vi "Transmit.vi"(8 "error in (no error)":errorcluster, 10 "Transfer Group in":refnum<class "Transfer Group.lvclass">, 11 "UDP Transceiver in":refnum<class "UDP Transceiver.lvclass">) -> (0 "error out":errorcluster, 2 "Transfer Group out":refnum<class "Transfer Group.lvclass">, 3 "UDP Transceiver out":refnum<class "UDP Transceiver.lvclass">)   [LabVIEW 2023, in "UDP.lvlib" / "UDP Transceiver.lvclass"]
uses:
  UDP Transceiver.lvclass
  Users/Public/Documents/National Instruments/NI VeriStand 2023/Custom Devices/Data Sharing Framework/Linux_x64/DSF Core.lvlibp/Classes/Transfer Group/Transfer Group.lvclass
  UDP Transceiver.lvclass/UDP Transceiver.ctl
  Write Datagram to Port.vi
  <vilib>/Utility/error.llb/Clear Errors.vi
  Users/Public/Documents/National Instruments/NI VeriStand 2023/Custom Devices/Data Sharing Framework/Linux_x64/DSF Core.lvlibp/Classes/Transfer/Get Active Buffer.vi
  Users/Public/Documents/National Instruments/NI VeriStand 2023/Custom Devices/Data Sharing Framework/Linux_x64/DSF Core.lvlibp/Classes/Buffer/Get Buffer Size.vi
  Users/Public/Documents/National Instruments/NI VeriStand 2023/Custom Devices/Data Sharing Framework/Linux_x64/DSF Core.lvlibp/Classes/Buffer/Read Buffer.vi
  Users/Public/Documents/National Instruments/NI VeriStand 2023/Custom Devices/Data Sharing Framework/Linux_x64/DSF Core.lvlibp/Classes/Buffer/Read Buffer 1D U8.vi
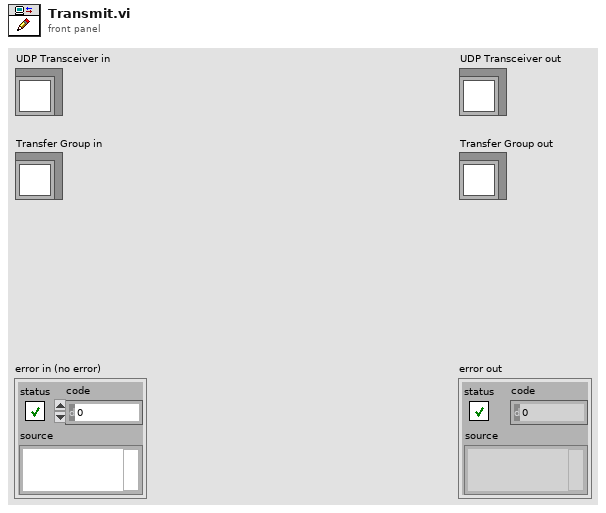
[diagram p1: front panel]
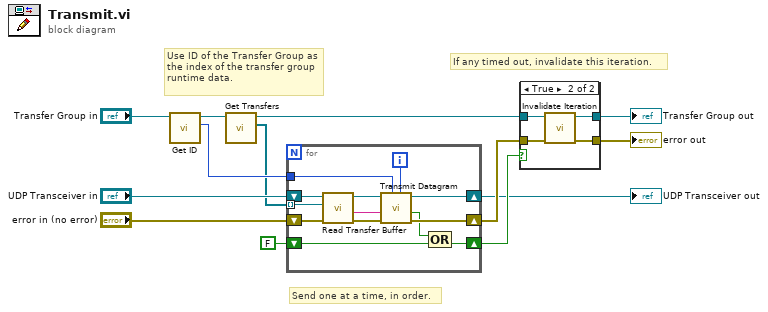
[diagram p0: block diagram]
diagram:
  # "If any timed out, invalidate this iteration."
  # "Send one at a time, in order."
  # "Use ID of the Transfer Group as the index of the transfer group runtime data."
  n1 = call "Get ID.vi"("Transfer Group in"="Transfer Group in") -> ("id"=w13:i32, "Transfer Group out"=w9:refnum<class "Transfer Group.lvclass">)  [unwired: 9 in]
  n2 = call "Get Transfers.vi"("Transfer Group in"=w9) -> ("Transfers"=w1:refnum<class "Transfer.lvclass">[], "Transfer Group out"=w7:refnum<class "Transfer Group.lvclass">)  [unwired: 9 in]
  n3 = for {
    shift-right: [w26] -> w5
    shift-left: "error in (no error)" -> [w18]
    shift-right: [w20] -> w2
    shift-left: "UDP Transceiver in" -> [w19]
    tunnel: w13 -> [w25]
    shift-right: [w21] -> w3
    shift-left: FALSE -> [w23]
    tunnel: w1 -> [w14] mode=indexing
    i -> [w24]
    n4 = call "Read Transfer Buffer.vi"("error in (no error)"=w18, "Transfer"=w14, "UDP Transceiver in"=w19) -> ("error out"=w15:errorcluster, "data"=w16:string, "UDP Transceiver out"=w17:refnum<class "UDP Transceiver.lvclass">)  [unwired: 6 in]
    n5 = call "Transmit Datagram.vi"("transfer id"=w24, "transfer group id"=w25, "error in (no error)"=w15, "transfer data"=w16, "UDP Transceiver in"=w17) -> ("error out"=w26:errorcluster, "timed out?"=w22:bool, "UDP Transceiver out"=w20:refnum<class "UDP Transceiver.lvclass">)  [unwired: 4 in]
    n6 = Compound Arithmetic op=OR(w22, w23) -> (w21:bool)
  }
  "UDP Transceiver out" <- w2
  n7 = case shown="True" w3 {
    tunnel: w7 -> [w27 w32]
    tunnel: [w27 w31] -> w6
    tunnel: w5 -> [w28 w30]
    tunnel: [w28 w29] -> w4
    frame False {
    }
    frame True {
      n8 = call "Invalidate Iteration.vi"("error in (no error)"=w30, "Transfer Group in"=w32) -> ("error out"=w29:errorcluster, "Transfer Group out"=w31:refnum<class "Transfer Group.lvclass">)  [unwired: 8 in]
    }
  }
  "error out" <- w4
  "Transfer Group out" <- w6
